vi "Get AO StringsAndValues.vi"(8 "error in (no error)":errorcluster, 11 "Instrument.Lockin in":refnum<class "Instrument.Lockin.lvclass">) -> (0 "error out":errorcluster, 2 "AO Strings and Values":cluster{string, i32}[](array[cluster]), 3 "Instrument.Lockin out":refnum<class "Instrument.Lockin.lvclass">)   [LabVIEW 2019, in "Instrument.Lockin.lvclass"]
uses:
  Instrument.Lockin.lvclass
  Instrument.Lockin.lvclass/Instrument.Lockin.ctl
  Instrument.DAQ/Instrument.DAQ.lvclass
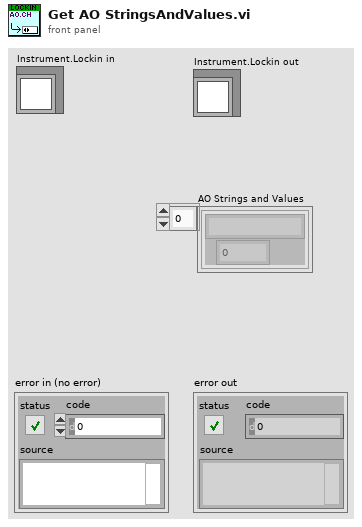
[diagram p1: front panel]
types:
  T1 = typedef "Instrument.DAQ.lvclass/AI.config-array.ctl" = T2[]
  T2 = typedef "Instrument.DAQ.lvclass/AI.config-cluster.ctl" = cluster{"AI.channels":tag, "AI.Coupling":T3, "AI.Range":T4, "input terminal configuration":i32, "DAQ Type":T5}
  T3 = typedef "Instrument.DAQ.lvclass/AI.coupling-enum.ctl" = u16
  T4 = typedef "Instrument.DAQ.lvclass/446xAI-enum.ctl" = enum16{"±0.316", "±1.00", "±3.16", "±10.0", "±31.6", "±42.4"}
  T5 = typedef "Instrument.DAQ.lvclass/DAQType-enum.ctl" = enum16{"None", "USB 4431", "PXI 446x"}
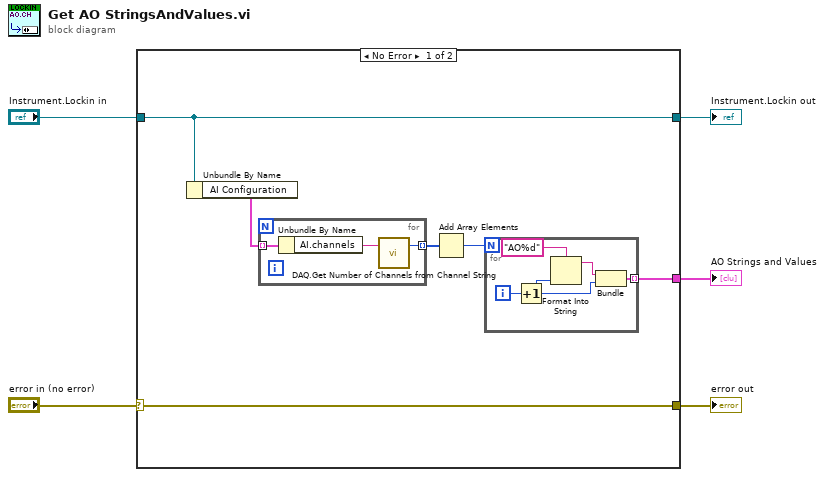
[diagram p0: block diagram]
diagram:
  n1 = case shown="No Error" "error in (no error)" {
    selector: "error in (no error)" -> [w6 w21]
    tunnel: "Instrument.Lockin in" -> [w7 w20]
    tunnel: [w8 _] -> w4
    tunnel: [w7 w20] -> w2
    tunnel: [w6 w21] -> w1
    frame No Error {
      n2 = Unbundle By Name(w7) -> ("AI Configuration"=w9:T1)
      n3 = for {
        tunnel: w9 -> [w14] mode=indexing
        tunnel: [w13] -> w10 mode=indexing
        n4 = Unbundle By Name(w14) -> ("AI.channels"=w12:tag)
        n5 = call "DAQ.Get Number of Channels from Channel String.vi"("Channels String"=w12) -> ("# channels"=w13:i32)  [unwired: 2 in]
      }
      n6 = Add Array Elements(numeric array=w10) -> (sum=w11:i32)
      n7 = for {
        N: w11 -> [_]
        tunnel: [w18] -> w8 mode=indexing
        i -> [w19]
        n8 = Increment(x=w19) -> (x+1=w17:i32)
        n9 = Format Into String(format string="AO%d", w17) -> (resulting string=w15:string)  [unwired: 2 in, 1 out]
        n10 = Bundle(w15, w17) -> (w18:cluster{string, i32})  [unwired: 1 in]
      }
    }
    frame Error {
    }
  }
  "AO Strings and Values" <- w4
  "Instrument.Lockin out" <- w2
  "error out" <- w1
